vi "Switch Determine Switch Type.vi"(4 "Switch Information":T2) -> (1 "Switch Type":T1)   [LabVIEW 2011]
uses:
  TypeDefs/Switch Instrument Info.ctl
  TypeDefs/Switch Type.ctl
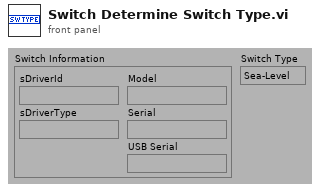
[diagram p1: front panel]
types:
  T1 = typedef "Switch Type.ctl" = enum16{"Sea-Level", "Simulator", "SI-0206-SW", "SI-0309-SW", "SI-0310-SW", "Front End"}
  T2 = typedef "Switch Instrument Info.ctl" = cluster{"sDriverId":string, "sDriverType":string, "Model":string, "Serial":string, "USB Serial":string}
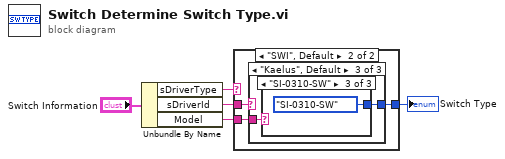
[diagram p0: block diagram]
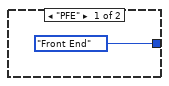
[diagram p2: hidden frame]
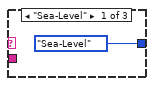
[diagram p3: hidden frame]
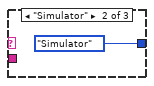
[diagram p4: hidden frame]
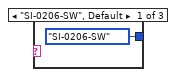
[diagram p5: hidden frame]
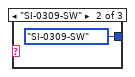
[diagram p6: hidden frame]
diagram:
  n1 = Unbundle By Name("Switch Information") -> ("sDriverType"=w1:string, "sDriverId"=w4:string, "Model"=w3:string)
  n2 = case shown="\"SWI\", Default" w1 {
    tunnel: w4 -> [_ w9]
    tunnel: w3 -> [_ w8]
    tunnel: [Switch_Type."Front End" ("Switch Type") w7] -> w2
    frame "PFE" {
    }
    frame "SWI", Default {
      n3 = case shown="\"Kaelus\", Default" w9 {
        tunnel: w8 -> [_ _ w13]
        tunnel: [Switch_Type."Sea-Level" ("Switch Type") Switch_Type."Simulator" ("Switch Type") w12] -> w7
        frame "Sea-Level" {
        }
        frame "Simulator" {
        }
        frame "Kaelus", Default {
          n4 = case shown="\"SI-0310-SW\"" w13 {
            tunnel: [Switch_Type."SI-0206-SW" ("Switch Type") Switch_Type."SI-0309-SW" ("Switch Type") Switch_Type."SI-0310-SW" ("Switch Type")] -> w12
            frame "SI-0206-SW", Default {
            }
            frame "SI-0309-SW" {
            }
            frame "SI-0310-SW" {
            }
          }
        }
      }
    }
  }
  "Switch Type" <- w2
